vi "FindFieldPosition.vi"(8 "error in (no error)":errorcluster, 9 "Field":T2, 10 "Board":T2[][](array[typedef])) -> (0 "error out":errorcluster, 2 "Position":T1)   [LabVIEW 2015, in "TronviewGame.lvlib" / "Board.lvclass"]
uses:
  Board.lvclass
  FieldState.ctl
  Position.ctl
panel:
  out "Found?":bool
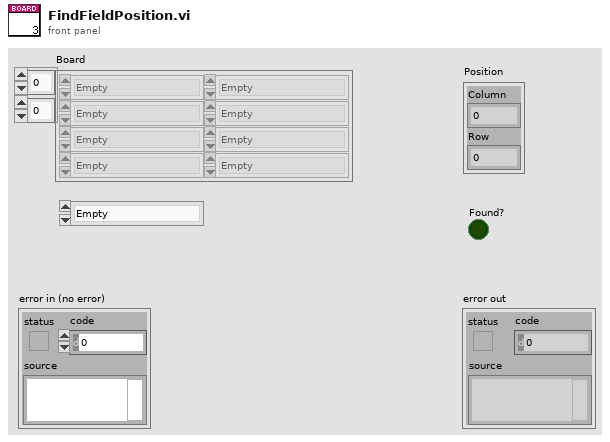
[diagram p1: front panel]
types:
  T1 = typedef "TronviewGame.lvlib/Board.lvclass/Position.ctl" = cluster{"Column":i32, "Row":i32}
  T2 = typedef "TronviewGame.lvlib/Board.lvclass/FieldState.ctl" = enum16{"Empty", "Blocked", "Player1Position", "Player2Postion", "Player1Marked", "Player2Marked"}
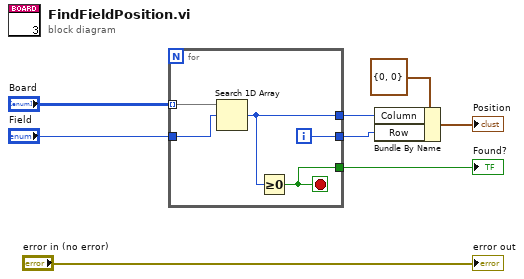
[diagram p0: block diagram]
diagram:
  n1 = for {
    tunnel: "Board" -> [w13] mode=indexing
    tunnel: "Field" -> [w12]
    tunnel: [w10] -> w3
    tunnel: [w11] -> w2
    tunnel: [w9] -> w1
    i -> [w11]
    stop <- w9 stop-if-true
    n2 = Search 1D Array(1D array=w13, element=w12) -> (index of element=w10:i32)  [unwired: 1 in]
    n3 = Greater Or Equal To 0?(x=w10) -> (x >= 0?=w9:bool)
  }
  "Found?" <- w1
  n4 = Bundle By Name(cluster=T1 {"Column"=0, "Row"=0} ("Position"), "Column"=w3, "Row"=w2) -> (→"Position":T1)
  "error out" <- "error in (no error)"
